vi "List Keys.vi"(7 "Section":string, 8 "error in (no error)":errorcluster, 11 "Ini Path in":path) -> (0 "error out":errorcluster, 1 "Section Found?":bool, 2 "Keys":string[](array[string]), 3 "Ini Path out":path)   [LabVIEW 2018, in "Cfg.lvlib"]
uses:
  Cfg.lvlib
  Action.ctl
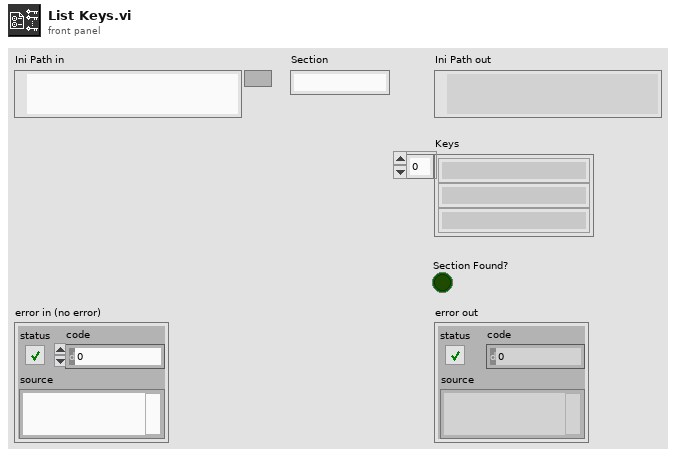
[diagram p1: front panel]
types:
  T1 = typedef "Cfg.lvlib/Action.ctl" = enum8{"noop", "new", "read_or_create", "read", "write", "remove", "keys", "sections", "remove_section", "import", "export", "get", "set", "pop", "add", "list", "list_sections", "pop_section"}
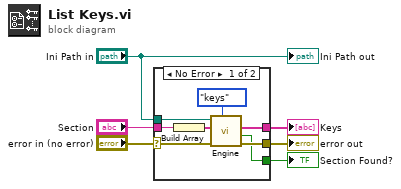
[diagram p0: block diagram]
diagram:
  n1 = case shown="No Error" "error in (no error)" {
    selector: "error in (no error)" -> [w14 w15]
    tunnel: "Ini Path in" -> [w12 _]
    tunnel: [w11 _] -> w4
    tunnel: [w10 w15] -> w3
    tunnel: "Section" -> [w9 _]
    tunnel: [w7 _] -> w1
    frame No Error {
      n2 = Build Array(w9) -> (w8:string[])
      n3 = call "Engine.vi"("Action"=Action."keys", "error in (no error)"=w14, "skvc in"=w8, "INI Path in"=w12) -> ("error out"=w10:errorcluster, "Found?"=w7:bool, "skvc out"=w11:string[])  [unwired: 4 in, 1 out]
    }
    frame Error {
    }
  }
  "error out" <- w3
  "Keys" <- w4
  "Section Found?" <- w1
  "Ini Path out" <- "Ini Path in"
